vi "Read Dew Point DBL.vi"(8 "error in":errorcluster, 10 "Source":string, 11 "Virtual NEO480 in":refnum<class "Virtual NEO480.lvclass">) -> (0 "error out":errorcluster, 1 "Time Stamp":timestamp format="%<%x %.3X>T", 2 "Dew Point":dbl, 3 "Virtual NEO480 out":refnum<class "Virtual NEO480.lvclass">)   [LabVIEW 2024, in "Virtual NEO480.lvclass"]
uses:
  Virtual NEO480.lvclass
  Virtual NEO480.lvclass/Virtual NEO480.ctl
  Source/DBC Communicator/DBC Communicator.lvclass
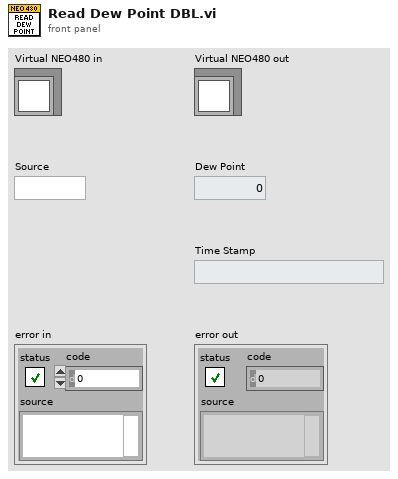
[diagram p1: front panel]
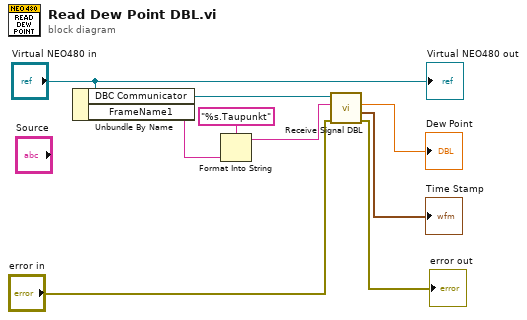
[diagram p0: block diagram]
diagram:
  n1 = Unbundle By Name("Virtual NEO480 in") -> ("DBC Communicator"=w6:refnum<class "DBC Communicator.lvclass">, "FrameName1"=w7:string)
  n2 = Format Into String(format string="%s.Taupunkt", w7) -> (resulting string=w5:string)  [unwired: 2 in, 1 out]
  n3 = call "Receive Signal DBL.vi"("error in"="error in", "Signal Name"=w5, "DBC Communication in"=w6) -> ("error out"=→"error out":errorcluster, "Time Stamp"=→"Time Stamp":timestamp, "Value"=→"Dew Point":dbl)  [unwired: 5 in, 1 out]
  "Virtual NEO480 out" <- "Virtual NEO480 in"
